vi "Close Bus Monitor.vi"(8 "error in (no error)":errorcluster, 11 "IBusMonitor In":refnum<class "IBusMonitor.lvclass">) -> (3 "IBusMonitor Out":refnum<class "IBusMonitor.lvclass">)   [LabVIEW 2019, in "MonitoredMediator.lvlib" / "IBusMonitor.lvclass"]
uses:
  <vilib>/gpm_packages/@cs/mva-core/Source/MonitoredMediator/IBusMonitor/IBusMonitor.lvclass
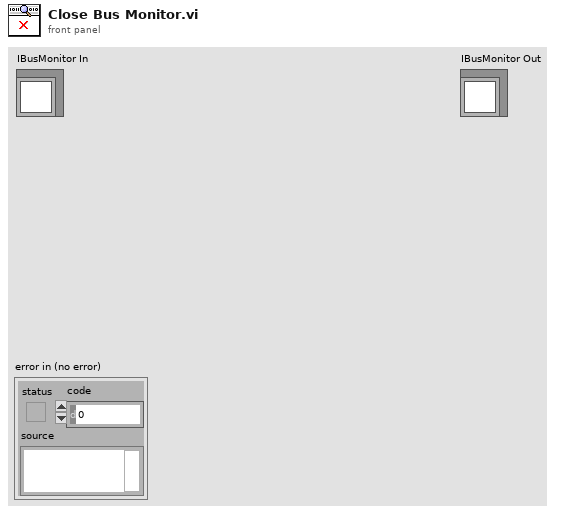
[diagram p1: front panel]
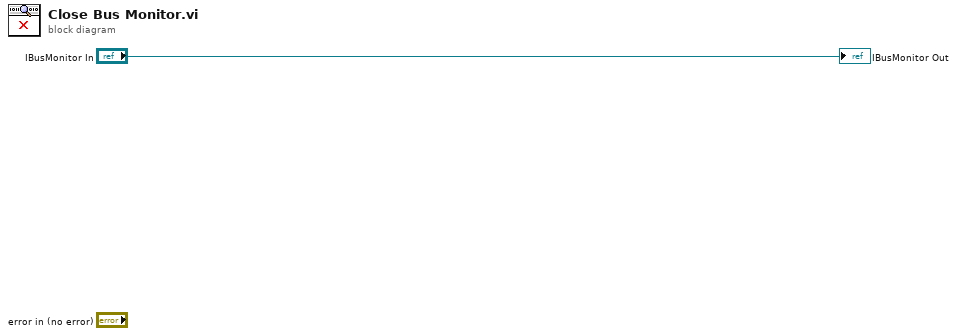
[diagram p0: block diagram]
diagram:
  "IBusMonitor Out" <- "IBusMonitor In"
